vi "test_Remove Custom Device.vi"(8 "error in (no error)":errorcluster, 11 "TestCase in":refnum<class "Scan Engine Unit Tests.lvclass">) -> (0 "error out":errorcluster, 3 "TestCase out":refnum<class "Scan Engine Unit Tests.lvclass">)   [LabVIEW 2017, in "Scan Engine Scripting API Custom Device Unit Tests.lvclass"]
uses:
  Scan Engine Scripting API Custom Device Unit Tests.lvclass
  Scan Engine Unit Tests.lvclass
  Type Defs/Main Settings.ctl
  <vilib>/addons/_JKI Toolkits/VI Tester/TestCase.llb/TestCase.lvclass
  Scripting/Scan Engine Scripting.lvlib
  Scan Engine Custom Device.lvlib
  C:/Program Files (x86)/National Instruments/LabVIEW 2017/vi.lib/addons/_JKI Toolkits/VI Tester/TestCase.llb/TestCase.lvclass
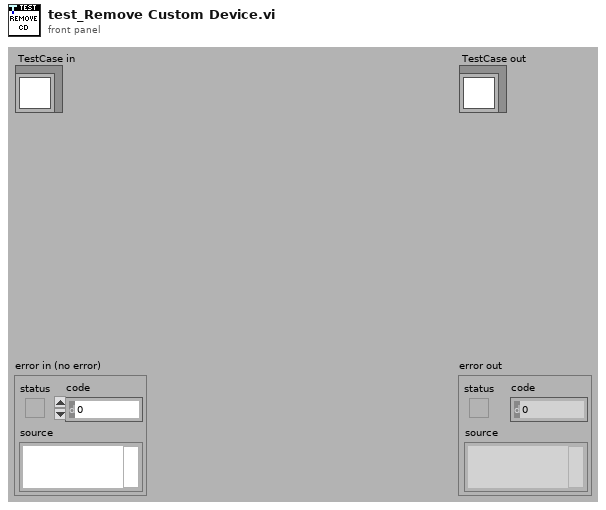
[diagram p1: front panel]
types:
  T1 = typedef "Scan Engine Custom Device.lvlib/Main Settings.ctl" = cluster{"sync to scan":bool, "scan engine decimation":u16, "delay after FPGA load (s)":u16}
  T2 = typedef "Custom Device API.lvlib/Custom Device Item Ref.ctl" = u64
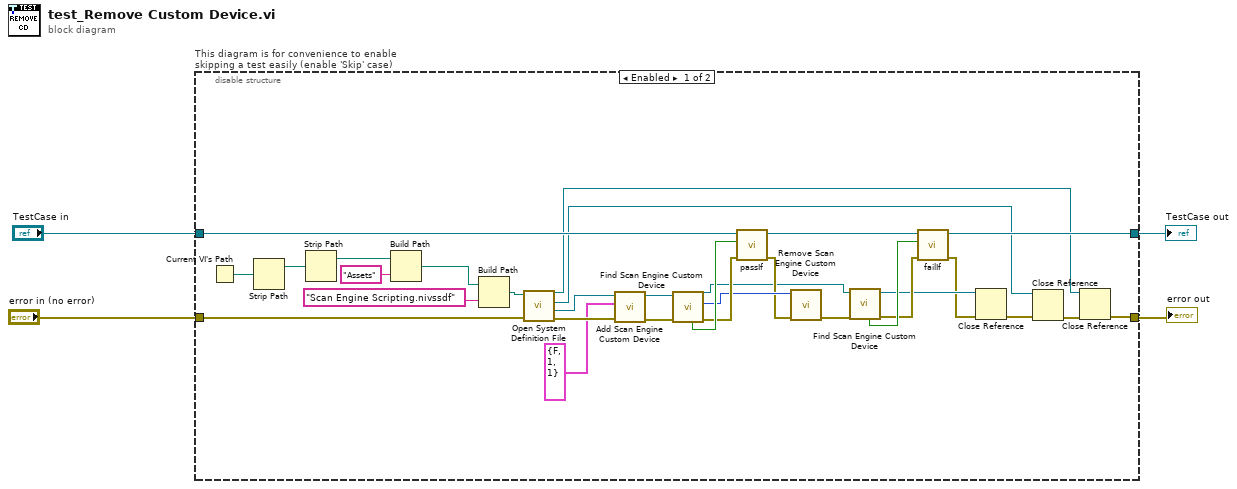
[diagram p0: block diagram]
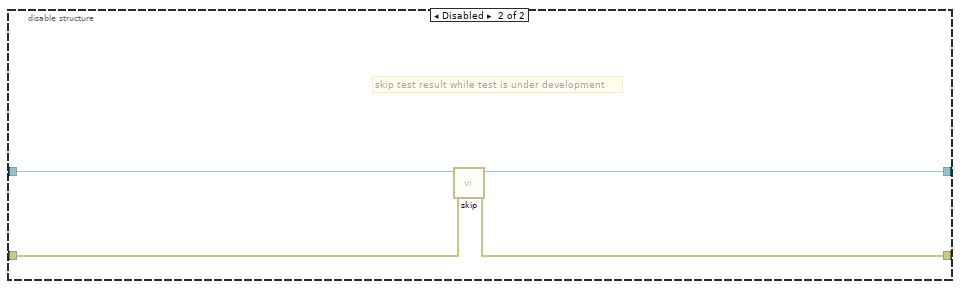
[diagram p2: hidden frame]
diagram:
  n1 = disable-structure "This diagram is for convenience to enable skipping a test easily (enable 'Skip' case)" shown="Enabled" {
    disable-tunnel: "TestCase in" -> [w24 w39]
    disable-tunnel: [w12 w37] -> w1
    disable-tunnel: [w5 w38] -> w3
    disable-tunnel: "error in (no error)" -> [w28 w36]
    frame Enabled {
      n2 = Current VI's Path() -> (path=w35:path)
      n3 = Strip Path(path=w35) -> (stripped path=w34:path)  [unwired: 1 out]
      n4 = Strip Path(path=w34) -> (stripped path=w33:path)  [unwired: 1 out]
      n5 = Build Path(base path=w33, name or relative path="Assets") -> (appended path=w31:path)
      n6 = Build Path(base path=w31, name or relative path="Scan Engine Scripting.nivssdf") -> (appended path=w29:path)
      n7 = call "Open System Definition File.vi"("error in"=w28, "path"=w29) -> ("error out"=w27:errorcluster, "target ref"=w25:refnum<k24>, "root ref"=w8:refnum<k24>, "system definition ref"=w6:refnum<k24>)  [unwired: 6 in]
      n8 = call "Add Scan Engine Custom Device.vi"("error in"=w27, "settings"=T1 {"sync to scan"=FALSE, "scan engine decimation"=1, "delay after FPGA load (s)"=1}, "target in"=w25) -> ("error out"=w23:errorcluster, "target out"=w22:refnum<k24>)  [unwired: 6 in, 1 out]
      n9 = call "Find Scan Engine Custom Device.vi"("error in"=w23, "target in"=w22) -> ("error out"=w20:errorcluster, "scan engine custom device ref"=w19:T2, "target out"=w16:refnum<k24>, "found"=w21:bool)  [unwired: 6 in]
      n10 = call-dynamic "passIf.vi"("error in (no error)"=w20, "pass"=w21, "TestCase in"=w24) -> ("error out"=w18:errorcluster, "TestCase out"=w14:refnum<class "Scan Engine Unit Tests.lvclass">)  [unwired: 7 in]
      n11 = call "Remove Scan Engine Custom Device.vi"("error in"=w18, "scan engine custom device ref in"=w19) -> ("error out"=w17:errorcluster)  [unwired: 9 in]
      n12 = call "Find Scan Engine Custom Device.vi"("error in"=w17, "target in"=w16) -> ("error out"=w13:errorcluster, "target out"=w11:refnum<k24>, "found"=w15:bool)  [unwired: 6 in, 1 out]
      n13 = call-dynamic "failIf.vi"("error in (no error)"=w13, "fail"=w15, "TestCase in"=w14) -> ("error out"=w10:errorcluster, "TestCase out"=w12:refnum<class "Scan Engine Unit Tests.lvclass">)  [unwired: 7 in]
      n14 = Close Reference(reference=w11, error in (no error)=w10) -> (error out=w9:errorcluster)
      n15 = Close Reference(reference=w8, error in (no error)=w9) -> (error out=w7:errorcluster)
      n16 = Close Reference(reference=w6, error in (no error)=w7) -> (error out=w5:errorcluster)
    }
    frame Disabled {
      # "skip test result while test is under development"
      n17 = call <vilib>:"skip.vi"("error in (no error)"=w36, "TestCase in"=w39) -> ("error out"=w38:errorcluster, "TestCase out"=w37:refnum<class "Scan Engine Unit Tests.lvclass">)  [unwired: 8 in]
    }
  }
  "error out" <- w3
  "TestCase out" <- w1
